vi "Loop Async.vi"(10 "ExecAnchor":refnum<class "ExecAnchor.lvclass">, 11 "Sequencing Control in":refnum<class "Sequencing Control.lvclass">) -> ()   [LabVIEW 2020, in "VolatusSeqGUI.lvlib" / "Sequencing Control.lvclass"]
uses:
  Sequencing Control.lvclass
  lv-exec-anchor/ExecAnchor/ExecAnchor.lvclass
  Sequencing Control.lvclass/Sequencing Control.ctl
  Volatus/VolatusAPI/VolatusAPI.lvclass
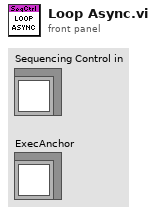
[diagram p1: front panel]
types:
  T1 = cluster{"Event Reg":refnum<event-registration>, "Event Reg":refnum<event-registration>}
  T2 = typedef "VolatusSeqGUI.lvlib/Sequencing Control.lvclass/Action.ctl" = enum16{"Details", "Load", "Unload", "Run", "Abort", "Unload All", "Abort All"}
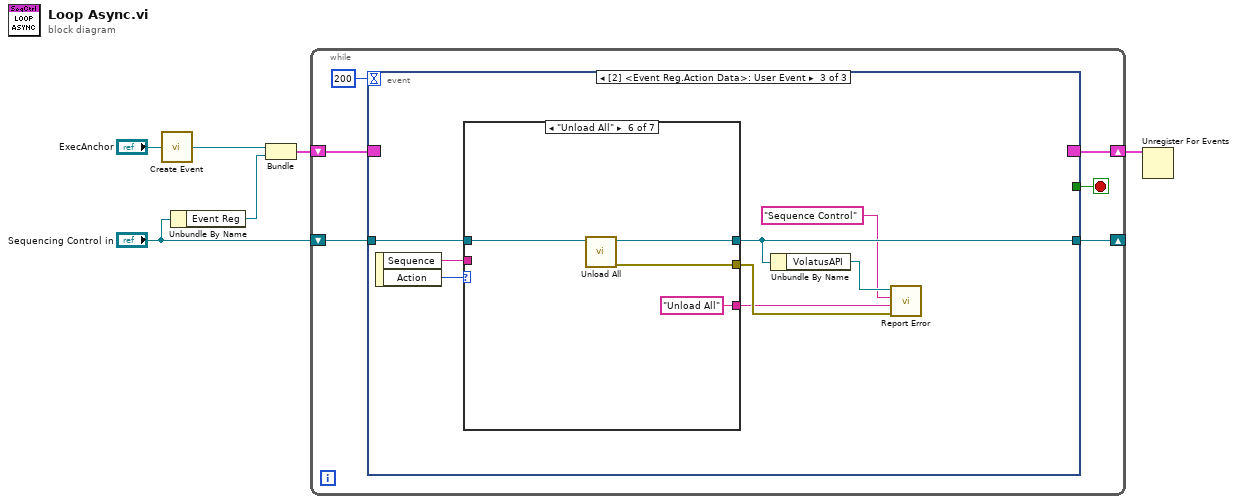
[diagram p0: block diagram]
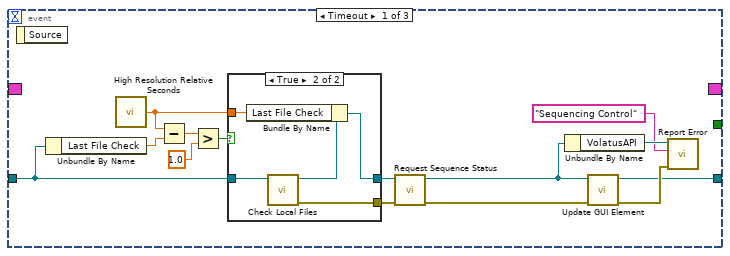
[diagram p2: hidden frame]
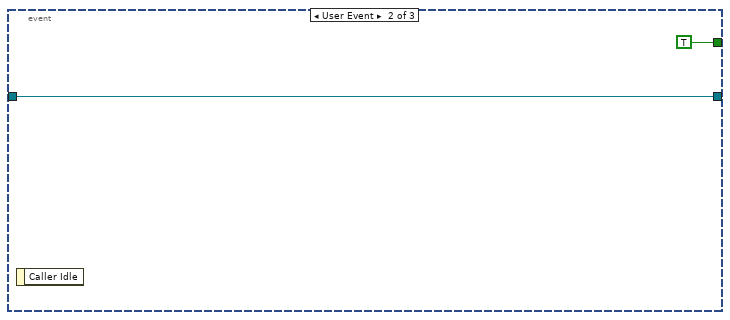
[diagram p4: hidden frame]
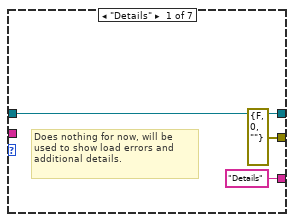
[diagram p5: hidden frame]
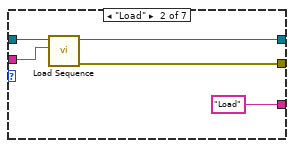
[diagram p6: hidden frame]
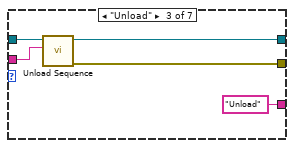
[diagram p7: hidden frame]
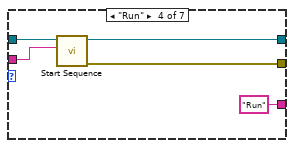
[diagram p8: hidden frame]
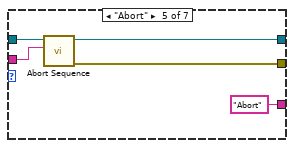
[diagram p9: hidden frame]
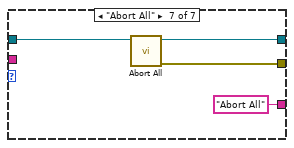
[diagram p10: hidden frame]
diagram:
  n1 = call "Create Event.vi"("ExecAnchor in"="ExecAnchor") -> ("Event Reg"=w5:refnum<event-registration>)  [unwired: 3 in, 1 out]
  n2 = Unbundle By Name("Sequencing Control in") -> ("Event Reg"=w1:refnum<event-registration>)
  n3 = Bundle("Event Reg"=w5, "Event Reg"=w1) -> (w2:T1)  [unwired: 1 in]
  n4 = while {
    shift-right: [w8] -> w4
    shift-left: w2 -> [w9]
    shift-right: [w10] -> _
    shift-left: "Sequencing Control in" -> [w11]
    stop <- w7 stop-if-true
    n5 = event shown="[2] <Event Reg.Action Data>: User Event" {
      selector: w9 -> [_ _ _]
      dyn-events: [_ _ _] -> w8
      timeout: 200 -> [_ _ _]
      tunnel: w11 -> [w22 w34 w42]
      tunnel: [w18 w34 w39] -> w10
      tunnel: [_ TRUE _] -> w7
      event Timeout {
        n6 = event-data() -> ()  [unwired: 1 in, 1 out]
        n7 = Unbundle By Name(w22) -> ("Last File Check"=w25:dbl)
        n8 = call <vilib>:"High Resolution Relative Seconds.vi"() -> ("relative seconds"=w20:dbl)
        n9 = Subtract(x=w20, y=w25) -> (x-y=w24:dbl)
        n10 = Greater?(x=w24, y=1.0) -> (0:w21:bool)
        n11 = case shown="True" w21 {
          tunnel: w22 -> [w27 w32]
          tunnel: w20 -> [_ w31]
          tunnel: [w27 w30] -> w19
          tunnel: [_ w28] -> w17
          frame False {
          }
          frame True {
            n12 = call "Check Local Files.vi"("Sequencing Control in"=w32) -> ("error out"=w28:errorcluster, "Sequencing Control out"=w29:refnum<class "Sequencing Control.lvclass">)  [unwired: 9 in]
            n13 = Bundle By Name(cluster=w29, "Last File Check"=w31) -> (w30:refnum<class "Sequencing Control.lvclass">)
          }
        }
        n14 = call "Request Sequence Status.vi"("error in (no error)"=w17, "Sequencing Control in"=w19) -> ("error out"=w13:errorcluster, "Sequencing Control out"=w16:refnum<class "Sequencing Control.lvclass">)  [unwired: 8 in]
        n15 = Unbundle By Name(w16) -> ("VolatusAPI"=w15:refnum<class "VolatusAPI.lvclass">)
        n16 = call "Update GUI Element.vi"("error in (no error)"=w13, "Sequencing Control in"=w16) -> ("error out"=w26:errorcluster, "Sequencing Control out"=w18:refnum<class "Sequencing Control.lvclass">)  [unwired: 8 in]
        n17 = call "Report Error.vi"("error in (no error)"=w26, "Context"="Sequencing Control", "VolatusAPI in"=w15) -> ()  [unwired: 7 in, 2 out]
      }
      event User Event {
        n18 = event-data() -> ()  [unwired: 1 in, 1 out]
      }
      event User Event {
        n19 = event-data() -> ("Sequence"=w40:string, "Action"=w41:T2)  [unwired: 1 in]
        n20 = case shown="\"Unload All\"" w41 {
          tunnel: w42 -> [w45 w50 w55 w59 w65 w69 w73]
          tunnel: [w45 w49 w54 w60 w64 w67 w71] -> w39
          tunnel: w40 -> [_ w48 w53 w58 w63 _ _]
          tunnel: [errorcluster {"status"=FALSE, "code"=0, "source"=""} ("error out") w47 w52 w57 w62 w66 w70] -> w37
          tunnel: ["Details" "Load" "Unload" "Run" "Abort" "Unload All" "Abort All"] -> w35
          frame "Details" {
            # "Does nothing for now, will be used to show load errors and additional details."
          }
          frame "Load" {
            n21 = call "Load Sequence.vi"("Sequence Name"=w48, "Sequencing Control in"=w50) -> ("error out"=w47:errorcluster, "Sequencing Control out"=w49:refnum<class "Sequencing Control.lvclass">)  [unwired: 8 in]
          }
          frame "Unload" {
            n22 = call "Unload Sequence.vi"("Sequence Name"=w53, "Sequencing Control in"=w55) -> ("error out"=w52:errorcluster, "Sequencing Control out"=w54:refnum<class "Sequencing Control.lvclass">)  [unwired: 8 in]
          }
          frame "Run" {
            n23 = call "Start Sequence.vi"("Sequence Name"=w58, "Sequencing Control in"=w59) -> ("error out"=w57:errorcluster, "Sequencing Control out"=w60:refnum<class "Sequencing Control.lvclass">)  [unwired: 8 in]
          }
          frame "Abort" {
            n24 = call "Abort Sequence.vi"("Sequence Name"=w63, "Sequencing Control in"=w65) -> ("error out"=w62:errorcluster, "Sequencing Control out"=w64:refnum<class "Sequencing Control.lvclass">)  [unwired: 8 in]
          }
          frame "Unload All" {
            n25 = call "Unload All.vi"("Sequencing Control in"=w69) -> ("error out"=w66:errorcluster, "Sequencing Control out"=w67:refnum<class "Sequencing Control.lvclass">)  [unwired: 9 in]
          }
          frame "Abort All" {
            n26 = call "Abort All.vi"("Sequencing Control in"=w73) -> ("error out"=w70:errorcluster, "Sequencing Control out"=w71:refnum<class "Sequencing Control.lvclass">)  [unwired: 9 in]
          }
        }
        n27 = Unbundle By Name(w39) -> ("VolatusAPI"=w38:refnum<class "VolatusAPI.lvclass">)
        n28 = call "Report Error.vi"("error in (no error)"=w37, "Message"=w35, "Context"="Sequence Control", "VolatusAPI in"=w38) -> ()  [unwired: 6 in, 2 out]
      }
    }
  }
  n29 = Unregister For Events(event registration refnum=w4) -> ()  [unwired: 1 in, 1 out]
